vi "test_Format Instrument String Command_Format array command(comma delimited, Type Cast).vi"(8 "error in (no error)":errorcluster, 11 "TestCase in":refnum<class "Instrument Addon Unit Tests.lvclass">) -> (0 "error out":errorcluster, 3 "TestCase out":refnum<class "Instrument Addon Unit Tests.lvclass">)   [LabVIEW 2020, in "Instrument Addon Unit Tests.lvclass"]
uses:
  Instrument Addon Unit Tests.lvclass
  Addon/Addon Shared/Types/Command Parameters.ctl
  Addon/Addon Shared/Types/Linked Channel Cluster.ctl
  Addon/Addon Shared/Types/Meta Data RT Configuration Cluster.ctl
  Addon/Addon Shared/Types/MetaData Parameters.ctl
  Addon/Addon Shared/Types/Protocol Data Type.ctl
  Addon/Addon Shared/Types/Metadata Channel Type.ctl
  Addon/Addon Shared/Types/Type Cast Type.ctl
  Addon/Addon Shared/Types/Endian.ctl
  Addon/Addon Engine/SubVIs/Format Numeric to String.vi
  <vilib>/addons/_JKI Toolkits/VI Tester/TestCase.llb/TestCase.lvclass
  Addon/Addon Engine/Instrument Addon Engine.lvlib
  Addon/Addon Shared/Instrument Addon Shared.lvlib
  C:/Program Files (x86)/National Instruments/LabVIEW 2020/vi.lib/addons/_JKI Toolkits/VI Tester/TestCase.llb/TestCase.lvclass
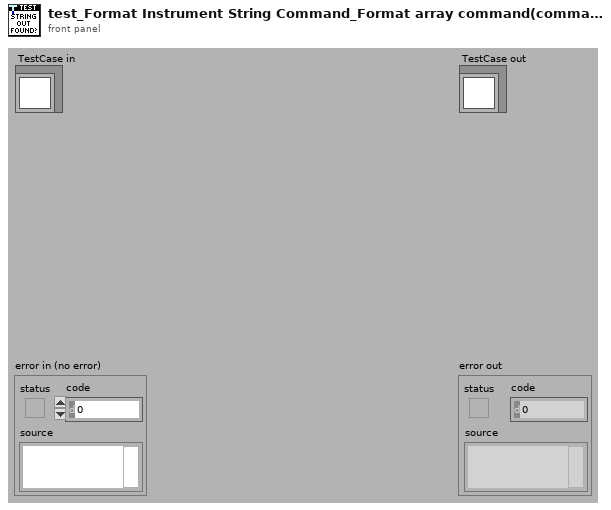
[diagram p1: front panel]
types:
  T1 = typedef "Instrument Addon Shared.lvlib/Meta Data RT Configuration Cluster.ctl" = cluster{"MetaData Parameters":T2, "Data Index":i32, "Data Length":i32}
  T2 = typedef "Instrument Addon Shared.lvlib/MetaData Parameters.ctl" = cluster{"Data Type":T3, "Channel Type":T4, "List":string[], "Format String":string, "Type":T5, "Delimiter":string, "Endian":T6}
  T3 = typedef "Instrument Addon Shared.lvlib/Protocol Data Type.ctl" = enum16{"Single Channel", "Array"}
  T4 = typedef "Instrument Addon Shared.lvlib/Metadata Channel Type.ctl" = enum16{"Enumerated List", "Format", "Type Cast"}
  T5 = typedef "Instrument Addon Shared.lvlib/Type Cast Type.ctl" = enum16{"DBL", "SGL", "U64", "U32", "U16", "U8", "I64", "I32", "I16", "I8"}
  T6 = typedef "Instrument Addon Shared.lvlib/Endian.ctl" = enum16{"Native", "Little", "Big"}
  T7 = typedef "Instrument Addon Shared.lvlib/Command Parameters.ctl" = cluster{"Command":string, "Linked Channels":T8[], "Pad":bool, "Length":u32, "Pad Value":u8}
  T8 = typedef "Instrument Addon Shared.lvlib/Linked Channel Cluster.ctl" = cluster{"Variable Name":string, "GUID":string}
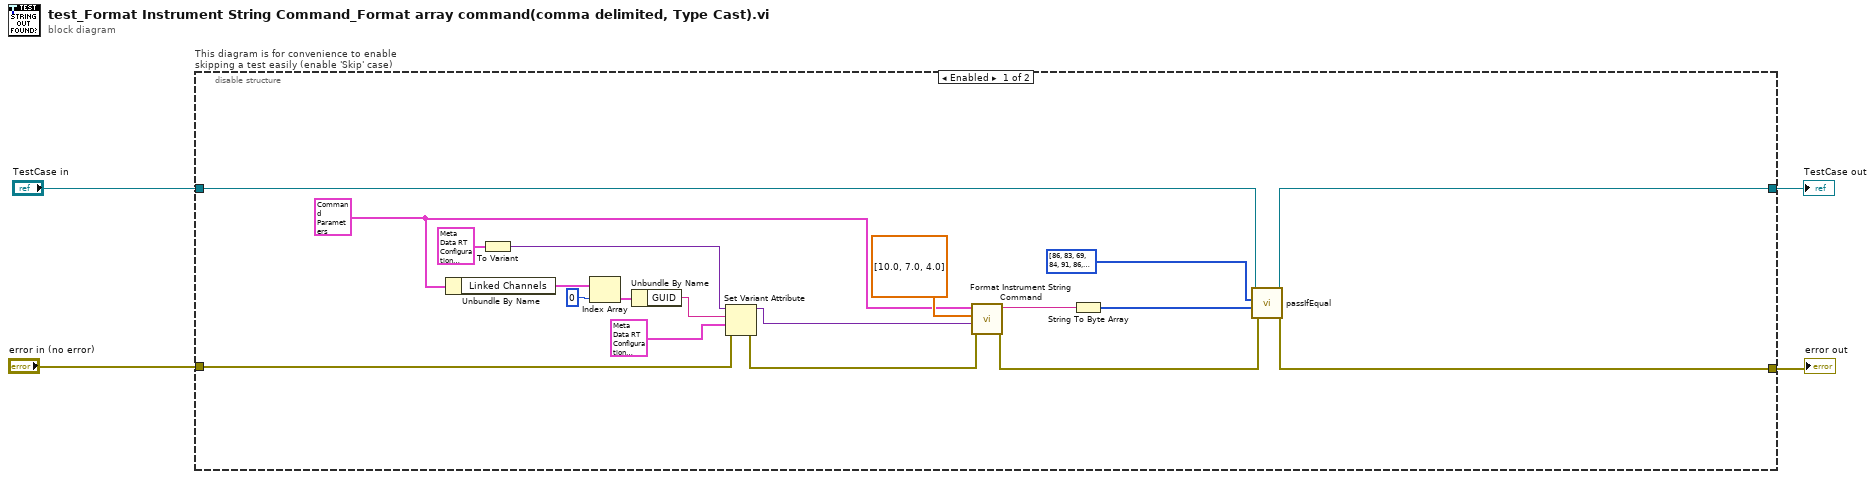
[diagram p0: block diagram]
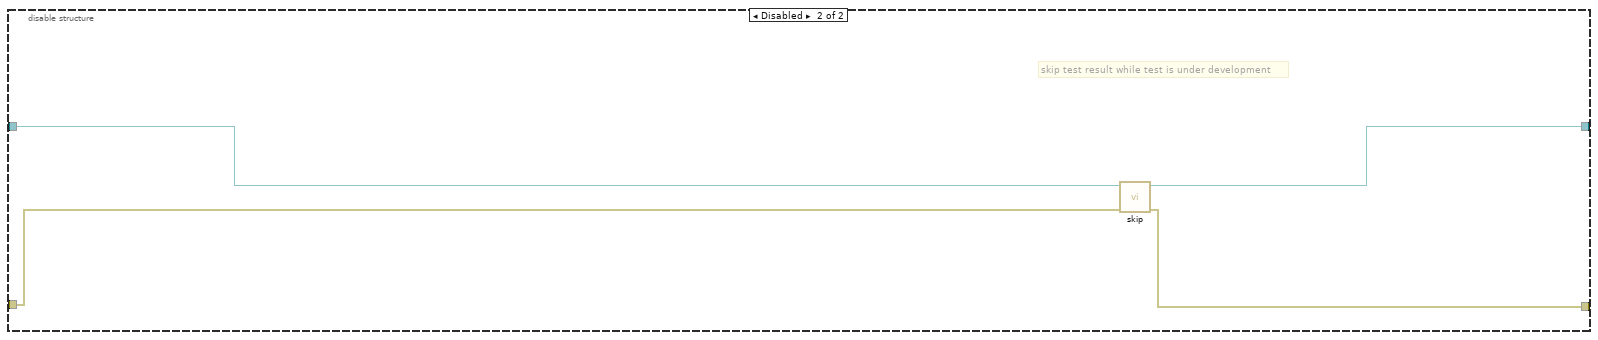
[diagram p2: hidden frame]
diagram:
  n1 = disable-structure "This diagram is for convenience to enable skipping a test easily (enable 'Skip' case)" shown="Enabled" {
    disable-tunnel: "TestCase in" -> [w23 w27]
    disable-tunnel: [w9 w25] -> w1
    disable-tunnel: [w22 w26] -> w3
    disable-tunnel: "error in (no error)" -> [w11 w24]
    frame Enabled {
      w17 = T7 {"Command"="VSET[VAR1]:[MetadataChannel]", "Linked Channels"=[{"Variable Name"="MetadataChannel", "GUID"="9428600d-6a85-43b8-aaac-a755da7e0c9b"}], "Pad"=FALSE, "Length"=0, "Pad Value"=0} ("Command Parameters")
      n2 = Unbundle By Name(w17) -> ("Linked Channels"=w16:T8[])
      n3 = To Variant(anything=T1 {"MetaData Parameters"={"Data Type"=enum."Single Channel", "Channel Type"=enum."Enumerated List", "List"=[], "Format String"="", "Type"=enum."DBL", "Delimiter"="", "Endian"=enum."Native"}, "Data Index"=0, "Data Length"=0}) -> (Variant=w20:variant)
      n4 = Index Array(array=w16, index=0) -> (element=w14:T8)
      n5 = Unbundle By Name(w14) -> ("GUID"=w13:string)
      n6 = Set Variant Attribute(Variant=w20, name=w13, value=T1 {"MetaData Parameters"={"Data Type"=enum."Array", "Channel Type"=enum."Type Cast", "List"=[], "Format String"="", "Type"=enum."DBL", "Delimiter"=",", "Endian"=enum."Native"}, "Data Index"=0, "Data Length"=3}, error in=w11) -> (Variant out=w19:variant, error out=w10:errorcluster)  [unwired: 1 out]
      n7 = call "Format Instrument String Command.vi"("error in (no error)"=w10, "MetaData Lookup in"=w19, "MetaData"=dbl[] [10.0, 7.0, 4.0], "Command Parameters"=w17) -> ("error out"=w8:errorcluster, "Command"=w7:string)  [unwired: 5 in, 1 out]
      n8 = String To Byte Array(string=w7) -> (unsigned byte array=w6:u8[])
      n9 = call-dynamic "passIfEqual.vi"("error in (no error)"=w8, "y"=w6, "x"=u8[] [86, 83, 69, 84, 91, 86, 65, 82, 49, 93, 58, 64, 36, 0, 0, 0, 0, 0, 0, 44, 64, 28, 0, 0, 0, 0, 0, 0, 44, 64, 16, 0, 0, 0, 0, 0, 0] ("unsigned byte array"), "TestCase in"=w23) -> ("error out"=w22:errorcluster, "TestCase out"=w9:refnum<class "Instrument Addon Unit Tests.lvclass">)  [unwired: 6 in]
    }
    frame Disabled {
      # "skip test result while test is under development"
      n10 = call <vilib>:"skip.vi"("error in (no error)"=w24, "TestCase in"=w27) -> ("error out"=w26:errorcluster, "TestCase out"=w25:refnum<class "Instrument Addon Unit Tests.lvclass">)  [unwired: 8 in]
    }
  }
  "error out" <- w3
  "TestCase out" <- w1
